vi "Execute.vi"(10 "Runnable":refnum<class "Runnable.lvclass">, 11 "Parallell Test Runner In":refnum<class "Parallell Test Runner.lvclass">) -> ()   [LabVIEW 2020, in "Parallell Test Runner.lvclass"]
uses:
  Parallell Test Runner.lvclass
  Core/Runnable/Runnable.lvclass
  Parallell Test Runner.lvclass/Parallell Test Runner.ctl
  Result Observer/Result Observer.lvclass
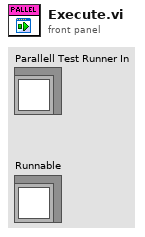
[diagram p1: front panel]
types:
  T1 = typedef "Result.lvlib/Result.ctl" = cluster{"Name":string, "Description":string, "Status":T2, "Result Type":T3, "Execution Time":dbl, "Data":cluster{"Expected":variant, "Actual":variant, "Delta":variant}}
  T2 = typedef "Result.lvlib/Status.ctl" = enum16{"", "Passed", "Failed", "Error", "Skipped", "Setup Error", "Broken", "Teardown Error"}
  T3 = typedef "Result.lvlib/Type.ctl" = enum16{"Test Case", "Test Suite", "Test Run", "Pass", "Fail", "Skip", "Pass if", "Fail if", "Pass if Error", "Fail if Error", "Pass if Equal", "Fail if Equal"}
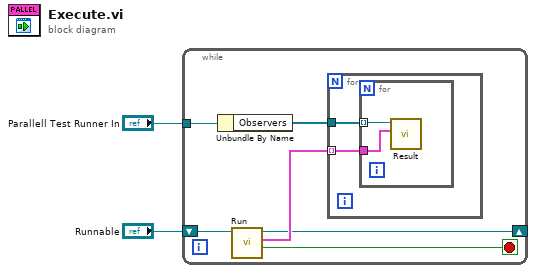
[diagram p0: block diagram]
diagram:
  n1 = while {
    shift-right: [w6] -> _
    shift-left: "Runnable" -> [w5]
    tunnel: "Parallell Test Runner In" -> [w4]
    stop <- w7 stop-if-true
    n2 = Unbundle By Name(w4) -> ("Observers"=w3:refnum<class "Result Observer.lvclass">[])
    n3 = call-dynamic "Run.vi"("Runnable In"=w5) -> ("Done?"=w7:bool, "Results"=w8:T1[], "Runnable Out"=w6:refnum<class "Runnable.lvclass">)  [unwired: 7 in, 1 out]
    n4 = for {
      tunnel: w8 -> [w9] mode=indexing
      tunnel: w3 -> [w10]
      n5 = for {
        tunnel: w10 -> [w12] mode=indexing
        tunnel: w9 -> [w11]
        n6 = call-dynamic "Result.vi"("Result"=w11, "Result Observer In"=w12) -> ()  [unwired: 9 in, 1 out]
      }
    }
  }
